vi "Teleop.vi"(10 "Match Info":T1={"Autonomous Elapsed Seconds"=0.0, "TeleOp Elapsed Seconds"=17.023, "Disabled Elapsed Seconds"=24.898, "Visited Autonomous"=FALSE, "Visited TeleOp"=TRUE, "Visited Disabled"=TRUE, "Autonomous Settings"={"Autonomous Style"=enum."Independent", "VI Refnum"=refnum}}, 11 "Call Context":T2=enum."Stop") -> ()   [LabVIEW 2018]
doc: "This VI is called for each TeleOp packet received from the DS where the robot is not disabled. It is often used to read from the joysticks and update I/O or to update setpoints for timed control loops. It should complete and return within 20 milliseconds or it may miss DS packets."
uses:
  <vilib>/Rock Robotics/WPI/DriverStation/WPI_DriverStationDerivedRobotMode.ctl
  <vilib>/Rock Robotics/WPI/DriverStation/WPI_DriverStationMatch Info.ctl
  <vilib>/Rock Robotics/WPI/ThirdParty/Phoenix-LabVIEW/Motor Controller/Controls/CTRE_Phoenix_MotorControl_ControlMode.ctl
  <vilib>/Rock Robotics/WPI/Utilities/WPI_GetSetVariantRefNum.vi
  <vilib>/Rock Robotics/Network Tables/NT Write Boolean Array.vi
  <vilib>/Rock Robotics/Network Tables/NT Write Numeric Array.vi
  <vilib>/Rock Robotics/Network Tables/NT Read Boolean.vi
  <vilib>/Rock Robotics/Network Tables/NT Read Number.vi
  <vilib>/Rock Robotics/WPI/ThirdParty/Phoenix-LabVIEW/Motor Controller/Get/CTRE_Phoenix_MotorController_GetOutputCurrent_Enhanced.vi
  <vilib>/Rock Robotics/WPI/ThirdParty/Phoenix-LabVIEW/Motor Controller/Get/CTRE_Phoenix_MotorController_GetVoltage.vi
panel:
  out "Current (Right)":dbl[](graph)
  out "Output Voltage":dbl[](graph)
  out "Current (Left)":dbl[](graph)
  in  "Max Turn":dbl(slide)=1.0 scale=0.0..1.0
  in  "Max Speed":dbl(slide)=1.0 scale=0.0..1.0
  out "Sample Slider 0":dbl(slide) scale=0.0..5.0
  out "Sample Boolean 1":bool
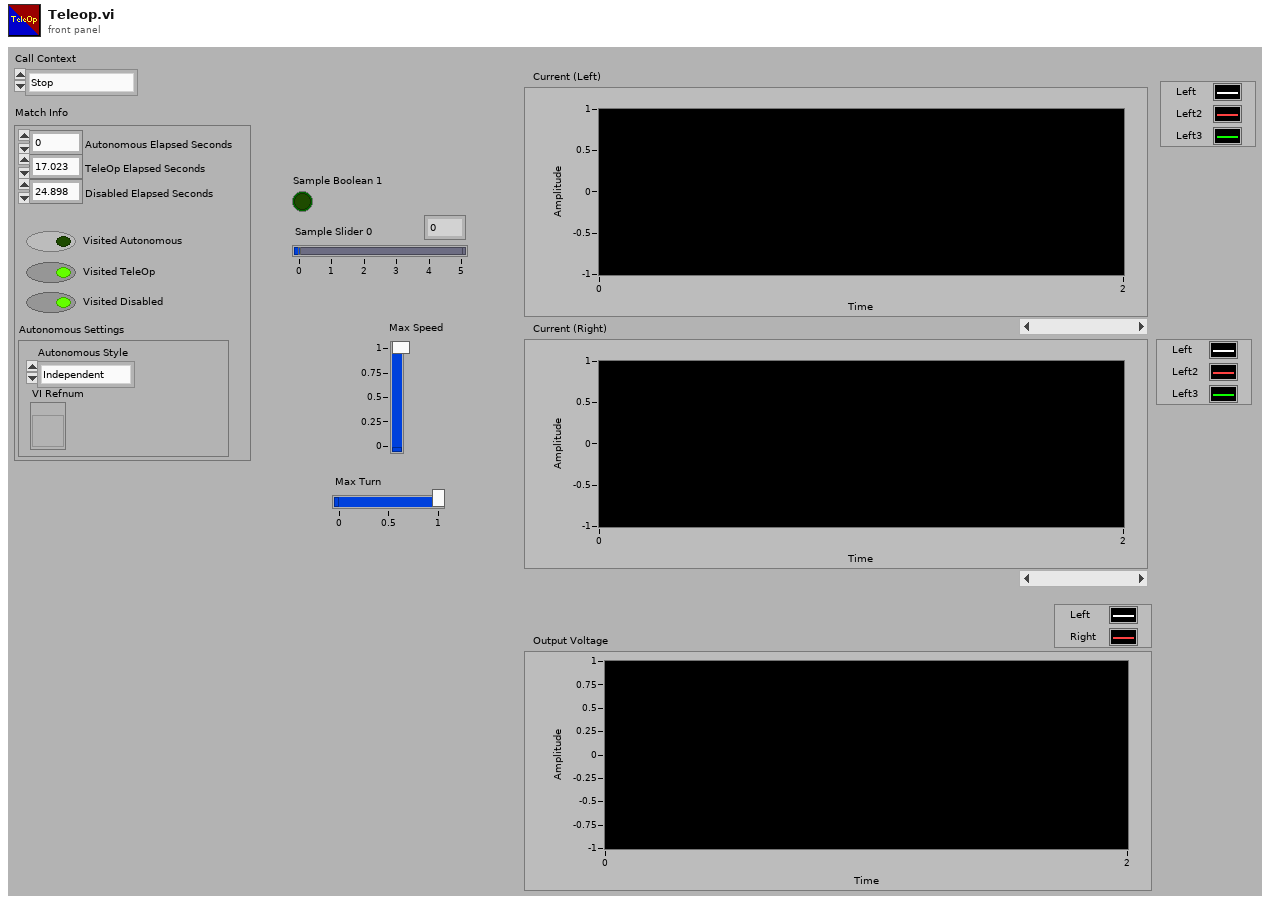
[diagram p1: front panel]
types:
  T1 = typedef "WPI_DriverStationMatch Info.ctl" = cluster{"Autonomous Elapsed Seconds":dbl, "TeleOp Elapsed Seconds":dbl, "Disabled Elapsed Seconds":dbl, "Visited Autonomous":bool, "Visited TeleOp":bool, "Visited Disabled":bool, "Autonomous Settings":cluster{"Autonomous Style":enum16{"Iterative", "Independent"}, "VI Refnum":refnum<vi>}}
  T2 = typedef "WPI_DriverStationDerivedRobotMode.ctl" = enum16{"Init", "Execute", "Stop"}
  T3 = typedef "CTRE_Phoenix_MotorControl_ControlMode.ctl" = u16
  T4 = typedef "WPI_JoystickDevRef.ctl" = cluster{"Device":T5}
  T5 = typedef "WPI_JoystickDeviceEnum.ctl" = enum16{"USB 0", "USB 1", "USB 2", "USB 3", "USB 4", "USB 5"}
  T6 = typedef "WPI_MotorControlDeviceRef.ctl" = cluster{"DeviceStatus":errorcluster, "Type":T7, "PWM":cluster{"PWM Channel":T8, "DeadBand":T9}, "CAN":cluster{"Device Number":u8, "SetOutput VI Ref":variant, "GetOutput VI Ref":variant, "Enable VI Ref":variant, "Disable VI Ref":variant, "Data":variant}, "Invert":bool, "DIO PWM":cluster{"PWM \"Enable\" Channel":T8, "DIOChannel":T10, "PWM Rate":dbl}}
  T7 = typedef "WPI_MotorControlType.ctl" = enum16{"PWM", "CAN", "DIO PWM"}
  T8 = typedef "FPGA_DIOPWMChannel.ctl" = enum8{"PWM 0", "PWM 1", "PWM 2", "PWM 3", "PWM 4", "PWM 5", "PWM 6", "PWM 7", "PWM 8", "PWM 9", "PWM MXP 0", "PWM MXP 1", "PWM MXP 2", "PWM MXP 3", "PWM MXP 4", "PWM MXP 5", "PWM MXP 6", "PWM MXP 7", "PWM MXP 8", "PWM MXP 9", "Invalid"}
  T9 = typedef "WPI_PWMDeadband.ctl" = cluster{"Name":string, "maxPositivePwm":i32, "minPositivePwm":i32, "centerPwm":i32, "maxNegativePwm":i32, "minNegativePwm":i32, "angularRange":u16}
  T10 = typedef "FPGA_DIOChannel.ctl" = enum8{"DIO 0", "DIO 1", "DIO 2", "DIO 3", "DIO 4", "DIO 5", "DIO 6", "DIO 7", "DIO 8", "DIO 9", "DIO MXP 0", "DIO MXP 1", "DIO MXP 2", "DIO MXP 3", "DIO MXP 4", "DIO MXP 5", "DIO MXP 6", "DIO MXP 7", "DIO MXP 8", "DIO MXP 9", "DIO MXP 10", "DIO MXP 11", "DIO MXP 12", "DIO MXP 13", "DIO MXP 14", "DIO MXP 15", "SPI Port CS1", "SPI Port CS2", "SPI Port CS3", "SPI Port MISO", "SPI Port MOSI", "Invalid"}
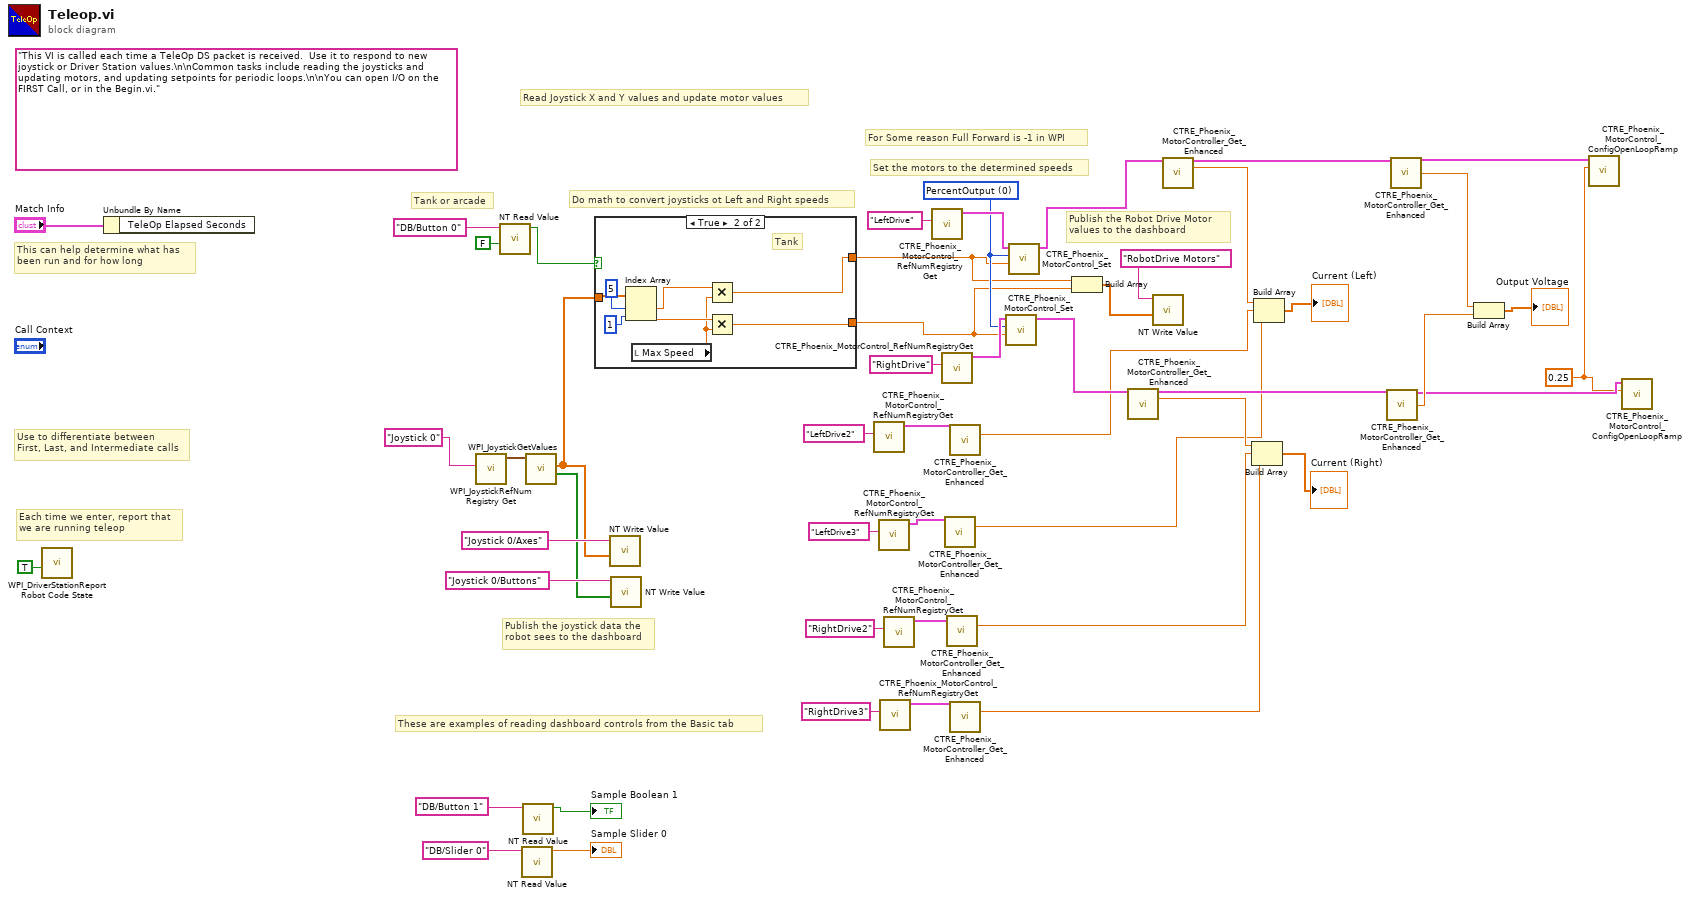
[diagram p0: block diagram]
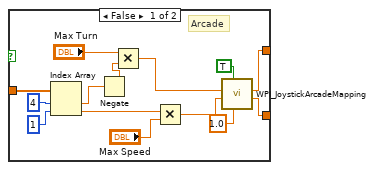
[diagram p2: hidden frame]
diagram:
  w15 = 0.25 ("secondsFromNeutralToFull")
  w30 = T3 0 items=["PercentOutput"=0, "Position"=1, "Velocity"=2, "Current"=3, "Follower"=5, "MotionProfile"=6, "MotionMagic"=7, "MotionProfileArc"=10, "Disabled"=15] ("Control Mode")
  (unwired) "This VI is called each time a TeleOp DS packet is received.  Use it to respond to new joystick or Driver Station values.\n\nCommon tasks include reading the joysticks and updating motors, and updating setpoints for periodic loops.\n\nYou can open I/O on the FIRST Call, or in the Begin.vi."
  # "For Some reason Full Forward is -1 in WPI"
  # "Set the motors to the determined speeds"
  # "Do math to convert joysticks ot Left and Right speeds"
  # "Tank or arcade"
  # "These are examples of reading dashboard controls from the Basic tab"
  # "Publish the Robot Drive Motor\nvalues to the dashboard"
  # "Publish the joystick data the\nrobot sees to the dashboard"
  # "Each time we enter, report that\nwe are running teleop"
  # "Use to differentiate between\nFirst, Last, and Intermediate calls"
  # "This can help determine what has\nbeen run and for how long"
  # "Read Joystick X and Y values and update motor values"
  n1 = call <vilib>:"WPI_DriverStationReport Robot Code State.vi"("TeleOp"=TRUE ("Autonomous")) -> ()  [unwired: 10 in, 1 out]
  n2 = Unbundle By Name("Match Info") -> ()  [unwired: 1 out]
  n3 = call <vilib>:"WPI_JoystickRefNum Registry Get.vi"("refnum name"="Joystick 0") -> ("JoystickDevRef"=w48:T4)  [unwired: 1 in, 9 out]
  n4 = call-poly <vilib>:"NT Read Value.vi"("Default Value"=FALSE, "Name"="DB/Button 0" ("refnum name")) -> ("Boolean"=w38:bool)  [unwired: 8 in, 1 out]
  n5 = call-poly <vilib>:"NT Read Value.vi"("Name"="DB/Slider 0" ("refnum name")) -> ("Numeric"=→"Sample Slider 0":dbl)  [unwired: 9 in, 1 out]
  n6 = call-poly <vilib>:"NT Read Value.vi"("Name"="DB/Button 1" ("refnum name")) -> ("Boolean"=→"Sample Boolean 1":bool)  [unwired: 9 in, 1 out]
  n7 = call <vilib>:"WPI_JoystickGetValues.vi"("JoystickDevRef"=w48) -> ("Buttons"=w44:bool[], "Axes"=w37:dbl[])  [unwired: 6 in, 3 out]
  n8 = case shown="True" w38 {
    tunnel: w37 -> [w64 w72]
    tunnel: [w55 w66] -> w28
    tunnel: [w54 w65] -> w27
    frame False {
      # "Arcade"
      n9 = Index Array(array=w64, index #1=4, index #2=1) -> (element #1=w52:dbl, element #2=w61:dbl)
      n10 = Negate(x=w52) -> (-x=w51:dbl)
      n11 = Multiply(x="Max Turn", y=w51) -> (x*y=w56:dbl)
      n12 = Multiply(x=w61, y="Max Speed") -> (x*y=w57:dbl)
      n13 = call <vilib>:"WPI_JoystickArcadeMapping.vi"("Max Output"=1.0, "Square Inputs"=TRUE, "Y axis value"=w57, "X axis value"=w56) -> ("Right Motor Value"=w54:dbl, "Left Motor Value"=w55:dbl)  [unwired: 6 in]
    }
    frame True {
      # "Tank"
      n14 = Index Array(array=w72, index #1=5, index #2=1) -> (element #1=w69:dbl, element #2=w68:dbl)
      n15 = local read "Max Speed"() -> (w67:dbl)
      n16 = Multiply(x=w69, y=w67) -> (x*y=w66:dbl)
      n17 = Multiply(x=w68, y=w67) -> (x*y=w65:dbl)
    }
  }
  n18 = call-poly <vilib>:"NT Write Value.vi"("Numeric Array"=w37, "Name"="Joystick 0/Axes") -> ()  [unwired: 9 in, 1 out]
  n19 = call-poly <vilib>:"NT Write Value.vi"("Boolean Array"=w44, "Name"="Joystick 0/Buttons") -> ()  [unwired: 9 in, 1 out]
  n20 = call <vilib>:"CTRE_Phoenix_MotorControl_RefNumRegistryGet.vi"("refnum name"="LeftDrive2") -> ("PhoenixMotorControlDevRef"=w10:T6)  [unwired: 9 in, 1 out]
  n21 = call <vilib>:"CTRE_Phoenix_MotorControl_RefNumRegistryGet.vi"("refnum name"="LeftDrive3") -> ("PhoenixMotorControlDevRef"=w9:T6)  [unwired: 9 in, 1 out]
  n22 = call <vilib>:"CTRE_Phoenix_MotorControl_RefNumRegistryGet.vi"("refnum name"="RightDrive3") -> ("PhoenixMotorControlDevRef"=w7:T6)  [unwired: 9 in, 1 out]
  n23 = call <vilib>:"CTRE_Phoenix_MotorControl_RefNumRegistryGet.vi"("refnum name"="RightDrive2") -> ("PhoenixMotorControlDevRef"=w8:T6)  [unwired: 9 in, 1 out]
  n24 = call <vilib>:"CTRE_Phoenix_MotorControl_RefNumRegistryGet.vi"("refnum name"="LeftDrive") -> ("PhoenixMotorControlDevRef"=w32:T6)  [unwired: 9 in, 1 out]
  n25 = call <vilib>:"CTRE_Phoenix_MotorControl_RefNumRegistryGet.vi"("refnum name"="RightDrive") -> ("PhoenixMotorControlDevRef"=w31:T6)  [unwired: 9 in, 1 out]
  n26 = call-poly <vilib>:"CTRE_Phoenix_MotorController_Get_Enhanced.vi"("PhoenixMotorControlDevRef"=w9) -> ("Output Current"=w2:dbl)  [unwired: 12 in, 2 out]
  n27 = call-poly <vilib>:"CTRE_Phoenix_MotorController_Get_Enhanced.vi"("PhoenixMotorControlDevRef"=w8) -> ("Output Current"=w5:dbl)  [unwired: 12 in, 2 out]
  n28 = call-poly <vilib>:"CTRE_Phoenix_MotorController_Get_Enhanced.vi"("PhoenixMotorControlDevRef"=w10) -> ("Output Current"=w3:dbl)  [unwired: 12 in, 2 out]
  n29 = call-poly <vilib>:"CTRE_Phoenix_MotorController_Get_Enhanced.vi"("PhoenixMotorControlDevRef"=w7) -> ("Output Current"=w4:dbl)  [unwired: 12 in, 2 out]
  n30 = call <vilib>:"CTRE_Phoenix_MotorControl_Set.vi"("Output"=w27, "Control Mode"=w30, "PhoenixMotorControlDevRef"=w31) -> ("PhoenixMotorControlDevRef"=w26:T6)  [unwired: 7 in, 1 out]
  n31 = call <vilib>:"CTRE_Phoenix_MotorControl_Set.vi"("Output"=w28, "Control Mode"=w30, "PhoenixMotorControlDevRef"=w32) -> ("PhoenixMotorControlDevRef"=w25:T6)  [unwired: 7 in, 1 out]
  n32 = Build Array(w28, w27) -> (w29:dbl[])
  n33 = call-poly <vilib>:"CTRE_Phoenix_MotorController_Get_Enhanced.vi"("PhoenixMotorControlDevRef"=w26) -> ("PhoenixMotorControlDevRef"=w20:T6, "Output Current"=w6:dbl)  [unwired: 12 in, 1 out]
  n34 = call-poly <vilib>:"NT Write Value.vi"("Numeric Array"=w29, "Name"="RobotDrive Motors") -> ()  [unwired: 9 in, 1 out]
  n35 = call-poly <vilib>:"CTRE_Phoenix_MotorController_Get_Enhanced.vi"("PhoenixMotorControlDevRef"=w25) -> ("PhoenixMotorControlDevRef"=w21:T6, "Output Current"=w23:dbl)  [unwired: 12 in, 1 out]
  n36 = Build Array(w6, w5, w4) -> (→"Current (Right)":dbl[])
  n37 = Build Array(w23, w3, w2) -> (→"Current (Left)":dbl[])
  n38 = call-poly <vilib>:"CTRE_Phoenix_MotorController_Get_Enhanced.vi"("PhoenixMotorControlDevRef"=w20) -> ("PhoenixMotorControlDevRef"=w16:T6, "Output Voltage"=w19:dbl)  [unwired: 10 in, 3 out]
  n39 = call-poly <vilib>:"CTRE_Phoenix_MotorController_Get_Enhanced.vi"("PhoenixMotorControlDevRef"=w21) -> ("PhoenixMotorControlDevRef"=w17:T6, "Output Voltage"=w18:dbl)  [unwired: 10 in, 3 out]
  n40 = Build Array(w18, w19) -> (→"Output Voltage":dbl[])
  n41 = call <vilib>:"CTRE_Phoenix_MotorControl_ConfigOpenLoopRamp.vi"("secondsFromNeutralToFull"=w15, "PhoenixMotorControlDevRef"=w17) -> ()  [unwired: 8 in, 2 out]
  n42 = call <vilib>:"CTRE_Phoenix_MotorControl_ConfigOpenLoopRamp.vi"("secondsFromNeutralToFull"=w15, "PhoenixMotorControlDevRef"=w16) -> ()  [unwired: 8 in, 2 out]
